vi "BRig_dataMTrig_warmup_CueSwitch.vi"() -> (2 "output_warmup_CueSwitch":i32)   [LabVIEW 2014]
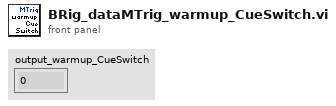
[diagram p1: front panel]
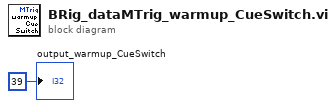
[diagram p0: block diagram]
diagram:
  "output_warmup_CueSwitch" <- 39 ("output_iBlock")
